vi "Check Rotate Done.vi"(8 "error in (no error)":errorcluster, 10 "start":u16=20032, 11 "phandle in":u32) -> (0 "error out":errorcluster)   [LabVIEW 2015]
uses:
  zauxdll-2014/zauxdll.lvlib
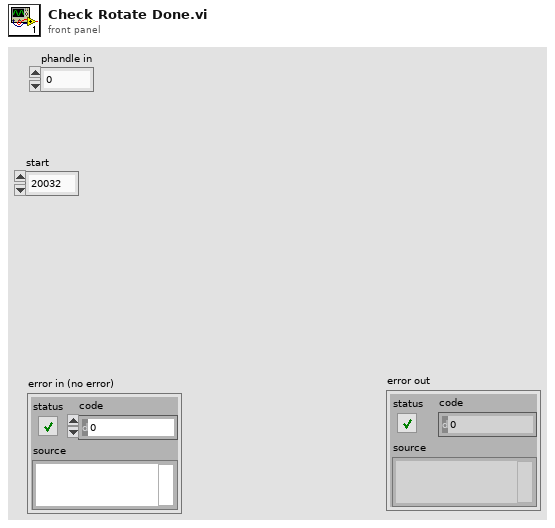
[diagram p1: front panel]
types:
  T1 = cluster{"unsigned byte array[0]":u8, "unsigned byte array[1]":u8, "unsigned byte array[2]":u8, "unsigned byte array[3]":u8, "unsigned byte array[4]":u8, "unsigned byte array[5]":u8, "unsigned byte array[6]":u8, "unsigned byte array[7]":u8, "unsigned byte array[8]":u8}
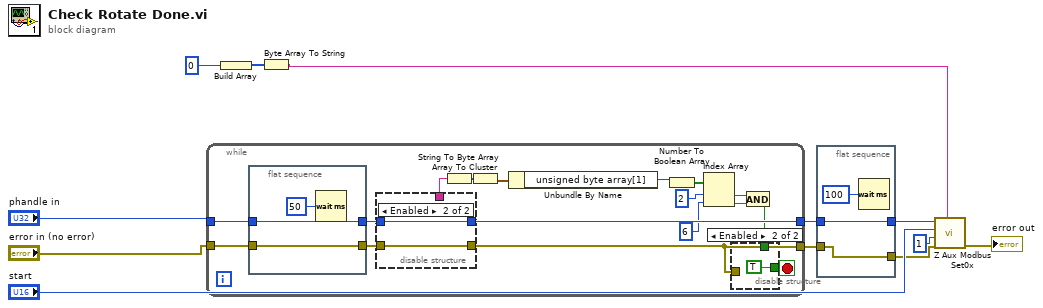
[diagram p0: block diagram]
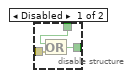
[diagram p2: hidden frame]
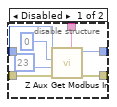
[diagram p3: hidden frame]
diagram:
  n1 = while {
    tunnel: "error in (no error)" -> [w16]
    tunnel: "phandle in" -> [w15]
    tunnel: [w23] -> w5
    tunnel: [w22] -> w3
    stop <- w24 stop-if-true
    n2 = flat-sequence {
      tunnel: w15 -> [w45]
      tunnel: [w45] -> w14
      tunnel: w16 -> [w43]
      tunnel: [w43] -> w13
      frame #0 {
        n3 = Wait (ms)(milliseconds to wait=u32 50) -> ()  [unwired: 1 out]
      }
    }
    n4 = disable-structure shown="Enabled" {
      disable-tunnel: [w38 _] -> w29
      disable-tunnel: [w37 w42] -> w23
      disable-tunnel: [w36 w41] -> w22
      disable-tunnel: w14 -> [w35 w41]
      disable-tunnel: w13 -> [w34 w42]
      frame Disabled {
        n5 = call "Z Aux Get Modbus In.vi"("error in (no error)"=w34, "ionumend"=23, "ionumfirst"=0, "handle"=w35) -> ("error out"=w37:errorcluster, "handle out"=w36:u32, "pValueList out"=w38:string)  [unwired: 4 in, 1 out]
      }
      frame Enabled {
      }
    }
    n6 = String To Byte Array(string=w29) -> (unsigned byte array=w28:u8[])
    n7 = Array To Cluster(array=w28) -> (cluster=w27:T1)
    n8 = Unbundle By Name(w27) -> ("unsigned byte array[1]"=w26:u8)
    n9 = Number To Boolean Array(number=w26) -> (Boolean array=w25:bool[])
    n10 = Index Array(array=w25, index #1=2, index #2=6) -> (element #1=w18:bool, element #2=w19:bool)
    n11 = And(x=w18, y=w19) -> (x .and. y?=w17:bool)
    n12 = disable-structure shown="Enabled" {
      disable-tunnel: [w32 TRUE] -> w24
      disable-tunnel: w23 -> [w31 _]
      disable-tunnel: w17 -> [w30 _]
      frame Disabled {
        n13 = Or(x=w30, y=w31) -> (x .or. y?=w32:bool)
      }
      frame Enabled {
      }
    }
  }
  n14 = Build Array(u32 0) -> (w12:u32[])
  n15 = Byte Array To String(unsigned byte array=w12) -> (string=w9:string)
  n16 = flat-sequence {
    tunnel: w5 -> [w48]
    tunnel: [w48] -> w4
    tunnel: w3 -> [w47]
    tunnel: [w47] -> w2
    frame #0 {
      n17 = Wait (ms)(milliseconds to wait=u32 100) -> ()  [unwired: 1 out]
    }
  }
  n18 = call "Z Aux Modbus Set0x.vi"("pdata"=w9, "error in (no error)"=w4, "inum"=u16 1, "start"="start", "handle"=w2) -> ("error out"=→"error out":errorcluster)  [unwired: 3 in, 3 out]
